vi "Export - Tx Packets.vi"(8 "error in (no error)":errorcluster, 11 "Device Item Ref in":T14 format="%.0x") -> (0 "error out":errorcluster, 3 "Tx Packets":T1 {"Tx Packet Data"."threadOptions"."pclDecimation" max=16 step=1; "Tx Packet Data"."threadOptions"."loopPeriod" max=16 step=1; "Tx Packet Data"."threadOptions"."targetPriority" min=-2 max=16 step=1; "Tx Packet Data"."threadOptions"."targetProcessor" min=-2 max=16 step=1; "Tx Packet Data"."Endianness" items=["big-endian"=0, "little-endian"=2]})   [LabVIEW 2019, in "UDP-Custom-Device System Explorer.lvlib"]
uses:
  UDP-Custom-Device System Explorer.lvlib
  <vilib>/NI VeriStand/Custom Device API/Custom Device Item Ref.ctl
  Types/XML - New/ImpExp - Tx Packets Data.ctl
  <vilib>/NI VeriStand/Custom Device API/Custom Device Item Info.ctl
  Types/XML - New/ImpExp - Tx Packet Data.ctl
  Shared/Types/Shared - Channel Data Type.ctl
  Shared/Types/Shared - Buffered.PacketInfo.ctl
  Shared/Types/Shared - Pointer Encoding.ctl
  Shared/Types/Shared - Receive Buffer Options.ctl
  Shared/Types/Shared - Transmit Buffer Options.ctl
  Shared/Types/Shared - Transmit Flag Options.ctl
  Shared/Types/Shared - Transmit Echo Options.ctl
  Types/Threading/Thread Configuration.ctl
  Types/Threading/Thread Sync Reference.ctl
  Shared/Types/Shared - Thread Management.ctl
  Shared/Constants.vi
  <vilib>/NI VeriStand/Custom Device API/Custom Device API.lvlib
  Property Accessors/Shared Section Accessors.lvlib
  Shared/UDP-Custom-Device Shared.lvlib
  <vilib>/NI VeriStand/Custom Device Tools/Custom Device Utility Library/Custom Device Utility Library.lvlib
  Property Accessors/Shared Packet Accessors.lvlib
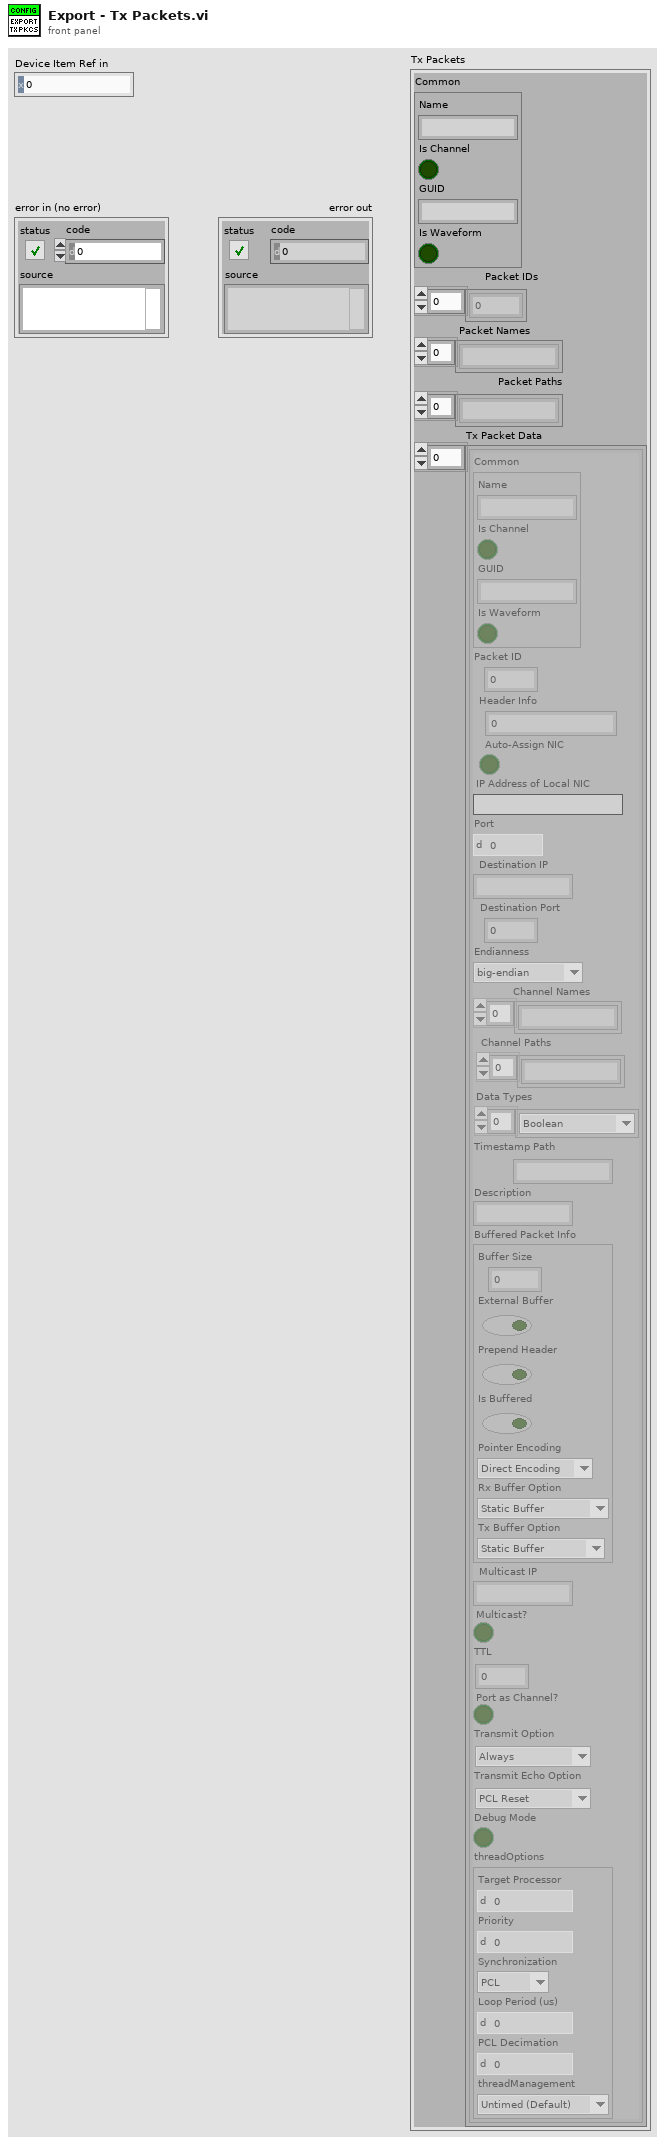
[diagram p1: front panel]
types:
  T1 = typedef "UDP-Custom-Device System Explorer.lvlib/ImpExp - Tx Packets Data.ctl" = cluster{"Common":T2, "Packet IDs":i32[], "Packet Names":string[], "Packet Paths":string[], "Tx Packet Data":T3[]}
  T2 = typedef "Custom Device API.lvlib/Custom Device Item Info.ctl" = cluster{"Name":string, "Is Channel":bool, "GUID":string, "Is Waveform":bool}
  T3 = typedef "UDP-Custom-Device System Explorer.lvlib/ImpExp - Tx Packet Data.ctl" = cluster{"Common":T2, "Packet ID":i32, "Header Info":u32, "Auto-Assign NIC":bool, "IP Address of Local NIC":string, "Port":u16, "Destination IP":string, "Destination Port":u16, "Endianness":u16, "Channel Names":string[], "Channel Paths":string[], "Data Types":T4[], "Timestamp Path":string, "Description":string, "Buffered Packet Info":T5, "Multicast IP":string, "Multicast?":bool, "TTL":u16, "Port as Channel?":bool, "Transmit Option":T9, "Transmit Echo Option":T10, "Debug Mode":bool, "threadOptions":T11}
  T4 = typedef "UDP-Custom-Device Shared.lvlib/Shared - Channel Data Type.ctl" = enum16{"Boolean", "Single", "Double", "I8", "I16", "I32", "I64", "U8", "U16", "U32", "U64"}
  T5 = typedef "UDP-Custom-Device Shared.lvlib/Shared - Buffered.PacketInfo.ctl" = cluster{"Buffer Size":i32, "External Buffer":bool, "Prepend Header":bool, "Is Buffered":bool, "Pointer Encoding":T6, "Rx Buffer Option":T7, "Tx Buffer Option":T8}
  T6 = typedef "UDP-Custom-Device Shared.lvlib/Shared - Pointer Encoding.ctl" = enum16{"Direct Encoding", "Conversion Encoding"}
  T7 = typedef "UDP-Custom-Device Shared.lvlib/Shared - Receive Buffer Options.ctl" = enum16{"Static Buffer", "Circular Buffer", "Circular Buffer + Size", "Internal Cache", "Internal Cache + Size", "Ping Pong", "Ping Pong + Size"}
  T8 = typedef "UDP-Custom-Device Shared.lvlib/Shared - Transmit Buffer Options.ctl" = enum16{"Static Buffer", "FIFO Buffer", "FIFO Buffer + Port"}
  T9 = typedef "UDP-Custom-Device Shared.lvlib/Shared - Transmit Flag Options.ctl" = enum16{"Always", "One-Shot", "Toggle"}
  T10 = typedef "UDP-Custom-Device Shared.lvlib/Shared - Transmit Echo Options.ctl" = enum16{"PCL Reset", "Counter", "Mirror"}
  T11 = typedef "UDP-Custom-Device System Explorer.lvlib/Thread Configuration.ctl" = cluster{"targetProcessor":i8, "targetPriority":i16, "Synchronization":T12, "loopPeriod":u32, "pclDecimation":u16, "threadManagement":T13}
  T12 = typedef "UDP-Custom-Device System Explorer.lvlib/Thread Sync Reference.ctl" = enum16{"PCL", "Async"}
  T13 = typedef "UDP-Custom-Device Shared.lvlib/Shared - Thread Management.ctl" = enum16{"Untimed (Default)", "Timed (High Priority)"}
  T14 = typedef "Custom Device API.lvlib/Custom Device Item Ref.ctl" = u64
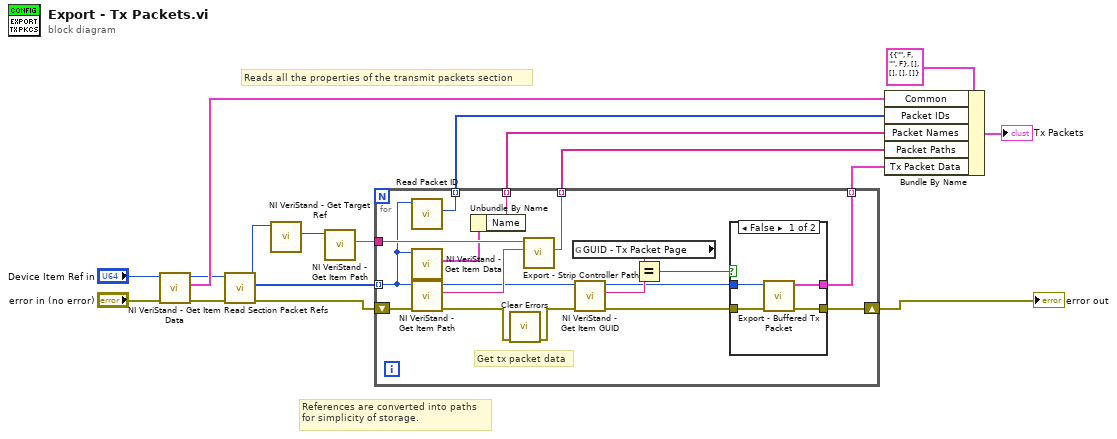
[diagram p0: block diagram]
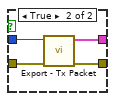
[diagram p2: hidden frame]
diagram:
  # "References are converted into paths\nfor simplicity of storage."
  # "Reads all the properties of the transmit packets section"
  n1 = call <vilib>:"NI VeriStand - Get Item Data.vi"("error in (no error)"="error in (no error)", "Item Ref in"="Device Item Ref in") -> ("error out"=w2:errorcluster, "Item Info"=w14:T2, "Item Ref out"=w3:T14)  [unwired: 6 in, 1 out]
  n2 = call "Read Section Packet Refs.vi"("error in (no error)"=w2, "Node Ptr"=w3) -> ("error out"=w12:errorcluster, "Dependent Node Refs"=w10:T14[], "Node Ptr out"=w7:T14)  [unwired: 7 in]
  n3 = call <vilib>:"NI VeriStand - Get Target Ref.vi"("Item Ref in"=w7) -> ("Target Ref"=w8:T14)  [unwired: 7 in, 3 out]
  n4 = call <vilib>:"NI VeriStand - Get Item Path.vi"("Item Ref in"=w8) -> ("Path"=w6:string)  [unwired: 7 in, 3 out]
  n5 = for {
    shift-right: [w34] -> w11
    shift-left: w12 -> [w35]
    tunnel: w10 -> [w28] mode=indexing
    tunnel: [w33] -> w9 mode=indexing
    tunnel: w6 -> [w31]
    tunnel: [w29] -> w5 mode=indexing
    tunnel: [w27] -> w4 mode=indexing
    tunnel: [w25] -> w1 mode=indexing
    # "Get tx packet data"
    n6 = call "Read Packet ID.vi"("Node Ptr"=w28) -> ("Packet ID"=w27:i32)  [unwired: 8 in, 2 out]
    n7 = call <vilib>:"NI VeriStand - Get Item Data.vi"("Item Ref in"=w28) -> ("Item Info"=w26:T2)  [unwired: 7 in, 3 out]
    n8 = call <vilib>:"NI VeriStand - Get Item Path.vi"("error in (no error)"=w35, "Item Ref in"=w28) -> ("error out"=w32:errorcluster, "Path"=w30:string, "Item Ref out"=w20:T14)  [unwired: 6 in, 1 out]
    n9 = Unbundle By Name(w26) -> ("Name"=w25:string)
    n10 = call <vilib>:"Clear Errors.vi"("error in (no error)"=w32) -> ("error out"=w22:errorcluster)  [unwired: 5 in, 1 out]
    n11 = call "Export - Strip Controller Path.vi"("Channel Path"=w30, "Controller Path"=w31) -> ("Stripped Path"=w29:string)  [unwired: 8 in, 1 out]
    n12 = global read "Constants.vi" "GUID - Tx Packet Page"() -> (w23:string)
    n13 = call <vilib>:"NI VeriStand - Get Item GUID.vi"("error in (no error)"=w22, "Item Ref in"=w20) -> ("error out"=w21:errorcluster, "GUID"=w24:string, "Item Ref out"=w19:T14)  [unwired: 7 in]
    n14 = Equal?(x=w23, y=w24) -> (x = y?=w18:bool)
    n15 = case shown="False" w18 {
      tunnel: [w37 w43] -> w34
      tunnel: [w36 w42] -> w33
      tunnel: w21 -> [w38 w41]
      tunnel: w19 -> [w39 w40]
      frame False {
        n16 = call "Export - Buffered Tx Packet.vi"("error in (no error)"=w38, "Device Item Ref in"=w39) -> ("error out"=w37:errorcluster, "Tx Packet"=w36:T3)  [unwired: 8 in]
      }
      frame True {
        n17 = call "Export - Tx Packet.vi"("error in (no error)"=w41, "Device Item Ref in"=w40) -> ("error out"=w43:errorcluster, "Tx Packet"=w42:T3)  [unwired: 8 in]
      }
    }
  }
  "error out" <- w11
  n18 = Bundle By Name(cluster=T1 {"Common"={"Name"="", "Is Channel"=FALSE, "GUID"="", "Is Waveform"=FALSE}, "Packet IDs"=[], "Packet Names"=[], "Packet Paths"=[], "Tx Packet Data"=[]} ("Tx Packets"), "Common"=w14, "Packet IDs"=w4, "Packet Names"=w1, "Packet Paths"=w5, "Tx Packet Data"=w9) -> (→"Tx Packets":T1)
